vi "Start Stop to Terminal Handles.vi"(8 "error in":errorcluster, 11 "Address Based Execution Unit Implementation in":refnum<class "Address Based Execution Unit.lvclass">) -> (0 "error out":errorcluster, 3 "Address Based Execution Unit Implementation out":refnum<class "Address Based Execution Unit.lvclass">)   [LabVIEW 2020, in "Ballard MIL-STD-1553 Engine.lvlib" / "Implementation.lvlib" / "Address Based Execution Unit.lvclass"]
uses:
  Implementation/Address Based Execution Unit/Address Based Execution Unit.lvclass
  <instrlib>/BTI1553Lib/BTI1553LV.lvlib
  Shared/Address.ctl
  Implementation/Address Based Execution Unit/Address Write Info.ctl
  Implementation/Execution Unit/Execution Unit.lvclass
  C:/dev/niveristand-ballard-milStd1553-custom-device/Source/Custom Device Support/Engine/Implementation/Execution Unit/Execution Unit.lvclass
  C:/dev/niveristand-ballard-milStd1553-custom-device/Source/Custom Device Support/Engine/Interfaces/Execution Unit/Execution Unit.lvclass
  C:/dev/niveristand-ballard-milStd1553-custom-device/Source/Custom Device Support/Engine/Implementation/Address Based Execution Unit/Address Based Execution Unit.lvclass
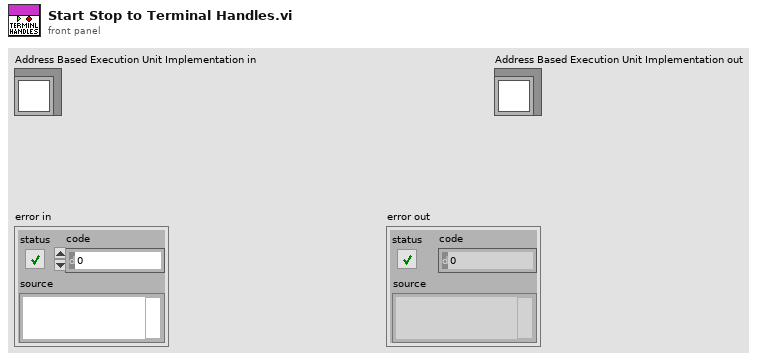
[diagram p1: front panel]
types:
  T1 = typedef "Ballard MIL-STD-1553 Engine.lvlib/Implementation.lvlib/Address Based Execution Unit.lvclass/Address Write Info.ctl" = cluster{"terminal address":T2, "terminal handle":u64}
  T2 = typedef "Address.ctl" = u16
  T3 = typedef "Ballard MIL-STD-1553 Engine.lvlib/Implementation.lvlib/Execution Unit.lvclass/1553 Start Stop Channel Handles.ctl" = cluster{"start stop handles":T4[]}
  T4 = typedef "Ballard MIL-STD-1553 Engine.lvlib/Implementation.lvlib/Execution Unit.lvclass/Start Stop Channel Handles.ctl" = cluster{"terminal address":T2, "start handle":T5, "stop handle":T5}
  T5 = typedef "Custom Device API.lvlib/Custom Device Item Ref.ctl" = u64
  T6 = typedef "Ballard MIL-STD-1553 Engine.lvlib/Custom Device.lvlib/Hardware Handles.ctl" = cluster{"core handle":u64, "core reader handle":u64, "channel handles":u64[]}
  T7 = typedef "1553 Channel.ctl" = cluster{"HW channel":u16, "terminals":T8[], "messages":T9[], "acyclic frame names":string[]}
  T8 = typedef "Terminal Name and Address.ctl" = cluster{"name":string, "terminal address":T2}
  T9 = typedef "Message Definition.ctl" = cluster{"name":string, "message type":T10, "endpoint Rx":T11, "endpoint Tx":T11, "mode code":u16, "number of words":u16, "parameters":cluster{"name":string, "default value":dbl, "unit":string, "parameter definition":T12}[], "create timestamp channel":bool}
  T10 = typedef "Message Type.ctl" = string
  T11 = typedef "Terminal Endpoint.ctl" = cluster{"terminal address":T2, "subaddress":T2}
  T12 = typedef "Parameter Definition.ctl" = cluster{"start index":i32, "size (bits)":i32, "encoding":enum16{"BNR", "BCD", "Discrete"}, "signed":bool, "multiplier":dbl, "offset":dbl}
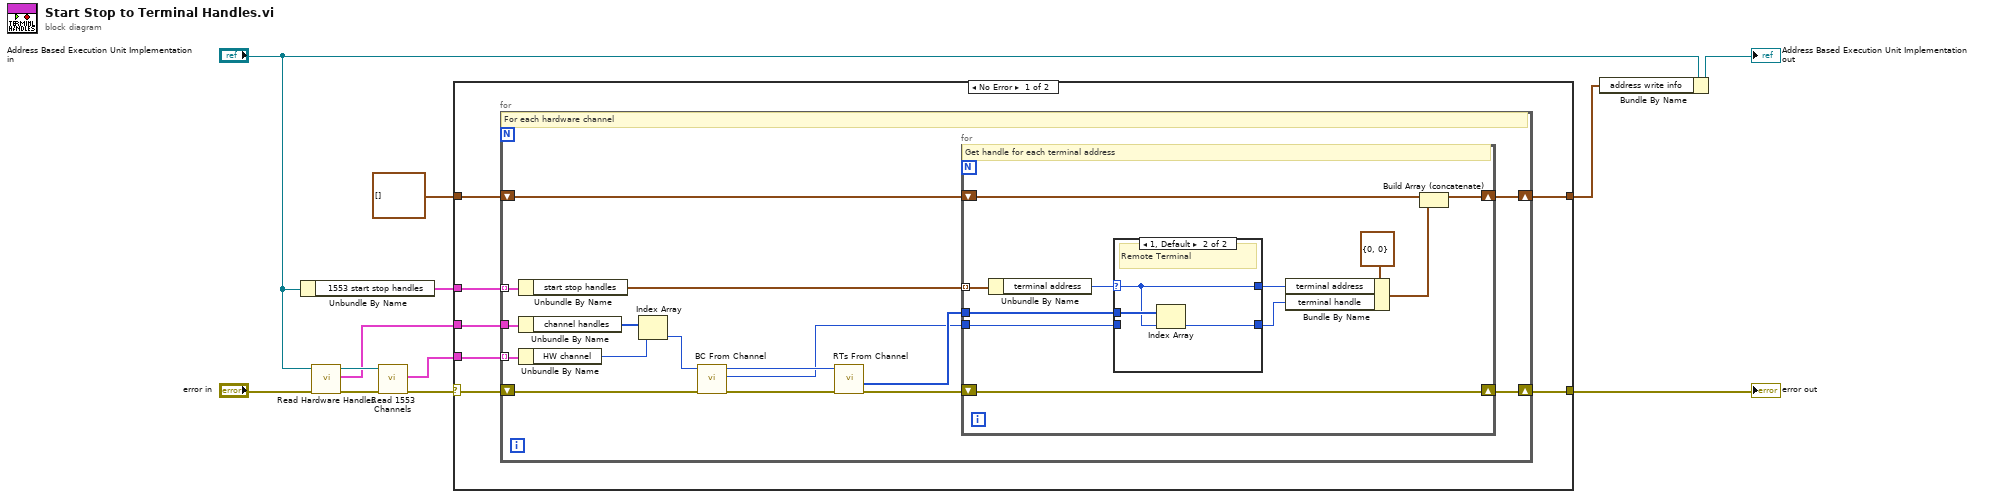
[diagram p0: block diagram]
diagram:
  n1 = Unbundle By Name("Address Based Execution Unit Implementation in") -> ("1553 start stop handles"=w4:T3[])
  n2 = call "Read Hardware Handles.vi"("error in"="error in", "Execution Unit in"="Address Based Execution Unit Implementation in") -> ("error out"=w8:errorcluster, "hardware handles"=w5:T6, "Execution Unit out"=w6:refnum<class "Address Based Execution Unit.lvclass">)  [unwired: 7 in]
  n3 = call "Read 1553 Channels.vi"("error in"=w8, "Execution Unit in"=w6) -> ("error out"=w9:errorcluster, "1553 channels"=w10:T7[])  [unwired: 7 in, 1 out]
  n4 = case shown="No Error" w9 {
    selector: w9 -> [w18 w52]
    tunnel: w10 -> [w15 _]
    tunnel: w5 -> [w19 _]
    tunnel: [w17 w52] -> w12
    tunnel: w4 -> [w16 _]
    tunnel: T1[] [] ("address write info") -> [w14 _]
    tunnel: [w13 _] -> w1
    frame No Error {
      n5 = for {
        tunnel: w15 -> [w35] mode=indexing
        tunnel: w19 -> [w34]
        shift-right: [w29] -> w17
        shift-left: w18 -> [w24]
        tunnel: w16 -> [w28] mode=indexing
        shift-right: [w20] -> w13
        shift-left: w14 -> [w21]
        # "For each hardware channel"
        n6 = Unbundle By Name(w28) -> ("start stop handles"=w27:T4[])
        n7 = Unbundle By Name(w34) -> ("channel handles"=w33:u64[])
        n8 = Unbundle By Name(w35) -> ("HW channel"=w32:u16)
        n9 = Index Array(array=w33, index=w32) -> (element=w26:u64)
        n10 = call <instrlib>:"BC From Channel.vi"("error in (no error)"=w24, "channel handle in"=w26) -> ("error out"=w23:errorcluster, "bus controller handle out"=w22:u64, "channel handle out"=w25:u64)  [unwired: 7 in]
        n11 = call <instrlib>:"RTs From Channel.vi"("error in (no error)"=w23, "channel handle in"=w25) -> ("error out"=w31:errorcluster, "remote terminal handles out"=w30:u64[])  [unwired: 6 in, 2 out]
        n12 = for {
          shift-right: [w46] -> w29
          shift-left: w31 -> [w46]
          tunnel: w30 -> [w44]
          tunnel: w27 -> [w45] mode=indexing
          tunnel: w22 -> [w42]
          shift-right: [w36] -> w20
          shift-left: w21 -> [w38]
          # "Get handle for each terminal address"
          n13 = Unbundle By Name(w45) -> ("terminal address"=w43:T2)
          n14 = case shown="1, Default" w43 {
            selector: w43 -> [w47 w49]
            tunnel: w44 -> [_ w51]
            tunnel: [w48 w50] -> w39
            tunnel: w42 -> [w48 _]
            tunnel: [w47 w49] -> w40
            frame 0 {
              # "Bus Controller"
            }
            frame 1, Default {
              # "Remote Terminal"
              n15 = Index Array(array=w51, index=w49) -> (element=w50:u64)
            }
          }
          n16 = Bundle By Name(cluster=T1 {"terminal address"=0, "terminal handle"=0} ("address write info"), "terminal address"=w40, "terminal handle"=w39) -> (w37:T1)
          n17 = Build Array (concatenate)(w38, w37) -> (w36:T1[])
        }
      }
    }
    frame Error {
    }
  }
  "error out" <- w12
  n18 = Bundle By Name(cluster="Address Based Execution Unit Implementation in", "address write info"=w1) -> (→"Address Based Execution Unit Implementation out":refnum<class "Address Based Execution Unit.lvclass">)
